vi "Write Message.vi"(8 "error in (no error)":errorcluster, 10 "Message":string, 11 "TCS_ACS in":refnum<class "TCS_ACS.lvclass">) -> (0 "error out":errorcluster, 3 "TCS_ACS out":refnum<class "TCS_ACS.lvclass">)   [LabVIEW 2018, in "TCS_ACS.lvclass"]
uses:
  TCS_ACS.lvclass
  TCS_ACS.lvclass/TCS_ACS.ctl
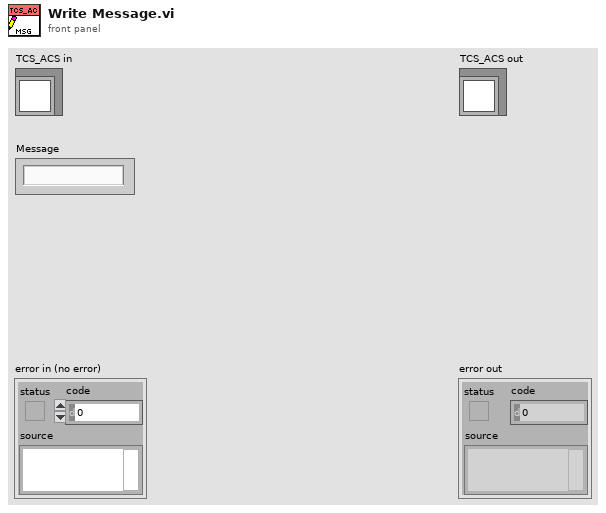
[diagram p1: front panel]
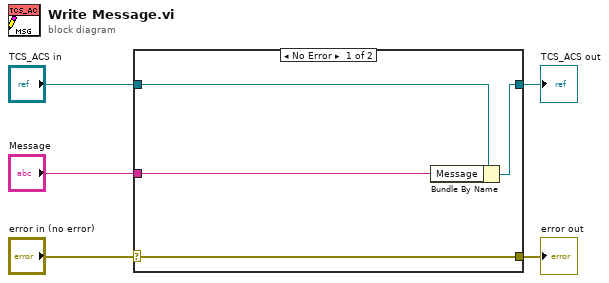
[diagram p0: block diagram]
diagram:
  n1 = case shown="No Error" "error in (no error)" {
    selector: "error in (no error)" -> [w9 w10]
    tunnel: [w9 w10] -> w4
    tunnel: [w7 w11] -> w2
    tunnel: "TCS_ACS in" -> [w8 w11]
    tunnel: "Message" -> [w6 _]
    frame No Error {
      n2 = Bundle By Name(cluster=w8, "Message"=w6) -> (w7:refnum<class "TCS_ACS.lvclass">)
    }
    frame Error {
    }
  }
  "error out" <- w4
  "TCS_ACS out" <- w2
